vi "21.Evd.8_Ask.2.vi"() -> ()   [LabVIEW 2025]
uses:
  <vilib>/Utility/file.llb/Write Delimited Spreadsheet (DBL).vi
panel:
  in  "Number of columns - measurements in Excel":dbl
  out "Tank digital":dbl
  out "Tank Analog":dbl(slide) scale=0.0..50000.0
  in  "Tank value":dbl(knob) scale=0.0..1000.0
  in  "stop":bool
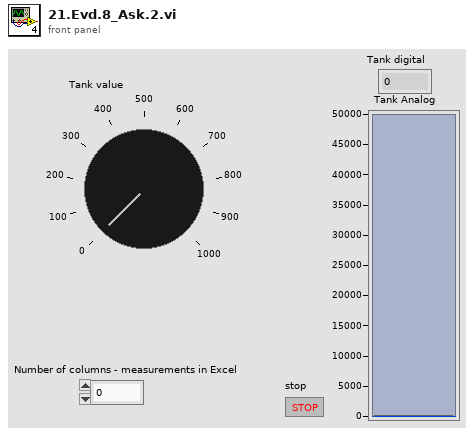
[diagram p1: front panel]
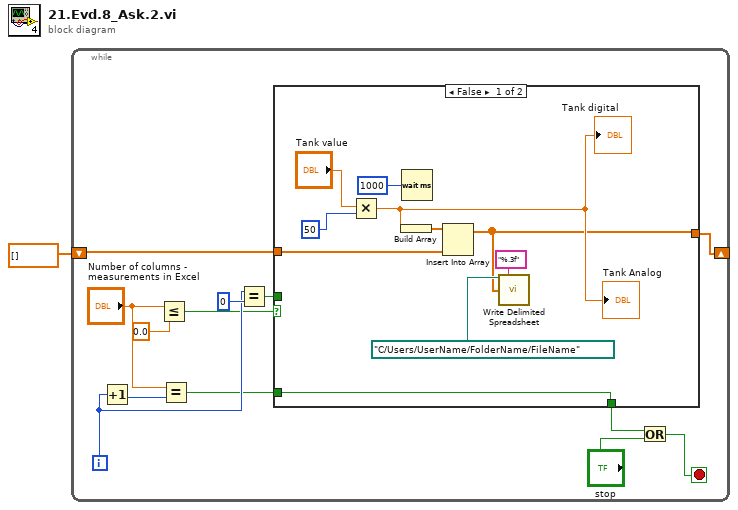
[diagram p0: block diagram]
diagram:
  n1 = while {
    shift-right: [w2] -> _
    shift-left: dbl[] [] -> [w3]
    i -> [w10]
    stop <- w11 stop-if-true
    n2 = Increment(x=w10) -> (x+1=w9:i32)
    n3 = Less Or Equal?(x="Number of columns - measurements in Excel", y=0.0) -> (x <= y?=w7:bool)
    n4 = Equal?(x="Number of columns - measurements in Excel", y=w9) -> (x = y?=w4:bool)
    n5 = Equal?(x=w10, y=0) -> (x = y?=w5:bool)
    n6 = case shown="False" w7 {
      tunnel: [w24 w25] -> w6
      tunnel: w5 -> [_ w25]
      tunnel: w4 -> [w24 _]
      tunnel: w3 -> [w19 _]
      tunnel: [w15 _] -> w2
      frame False {
        n7 = Multiply(x="Tank value", y=50) -> (x*y=w21:dbl)
        "Tank Analog" <- w21
        "Tank digital" <- w21
        n8 = Build Array(w21) -> (w22:dbl[])
        n9 = Wait (ms)(milliseconds to wait=u32 1000) -> ()  [unwired: 1 out]
        n10 = Insert Into Array(array=w22, new element=w19) -> (w15:dbl[])  [unwired: 1 in]
        n11 = call-poly <vilib>:"Write Delimited Spreadsheet.vi"("file path (dialog if empty)"=path "C:/Users/UserName/FolderName/FileName", "format (%.3f)"="%.3f", "1D data"=w15) -> ()  [unwired: 11 in, 2 out]
      }
      frame True {
      }
    }
    n12 = Or(x=w6, y="stop") -> (x .or. y?=w11:bool)
  }
